vi "Square Wave PtByPt.vi"(0 "amplitude":dbl=1.0 format="%0.2f", 1 "frequency":dbl=1.0 format="%0.2f", 2 "phase":dbl format="%0.2f", 3 "time":dbl format="%0.2f", 4 "duty cycle (%)":dbl=50.0 format="%0.2f") -> (5 "square wave":dbl format="%0.2f")   [LabVIEW 2017, in "NI_PtbyPt.lvlib"]
doc: "Generates a square wave point by point."
uses:
  <vilib>/ptbypt/NI_PtbyPt.lvlib
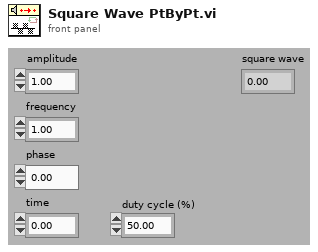
[diagram p1: front panel]
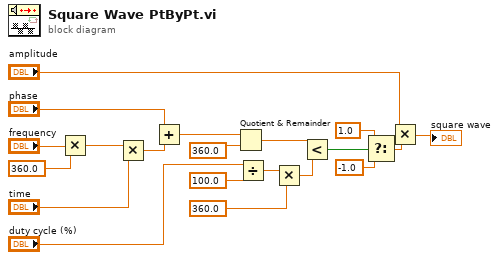
[diagram p0: block diagram]
diagram:
  n1 = Multiply(x="frequency", y=360.0 ("x")) -> (x*y=w20:dbl)
  n2 = Multiply(x=w20, y="time") -> (x*y=w13:dbl)
  n3 = Add(x="phase", y=w13) -> (x+y=w12:dbl)
  n4 = Quotient & Remainder(x=w12, y=360.0) -> (x-y*floor(x/y)=w4:dbl)  [unwired: 1 out]
  n5 = Divide(x="duty cycle (%)", y=100.0) -> (x/y=w10:dbl)
  n6 = Multiply(x=w10, y=360.0) -> (x*y=w9:dbl)
  n7 = Less?(x=w4, y=w9) -> (x < y?=w8:bool)
  n8 = Select(t=1.0, s=w8, f=-1.0) -> (s? t:f=w5:dbl)
  n9 = Multiply(x="amplitude", y=w5) -> (x*y=→"square wave":dbl)
